vi "DBL to String (3dp).vi"(11 "Number":dbl) -> (3 "String":string)   [LabVIEW 2018, in "Main.lvlib"]
uses:
  Main.lvlib
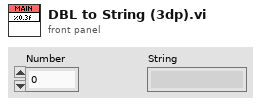
[diagram p1: front panel]
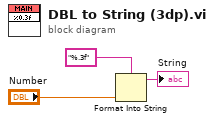
[diagram p0: block diagram]
diagram:
  n1 = Format Into String(format string="%.3f", "Number") -> (resulting string=→"String":string)  [unwired: 2 in, 1 out]
